vi "Test Report Contains Failed Test Result.vi"(8 "error in (no error)":errorcluster, 11 "Text Report Test in":refnum<class "Text Report Test.lvclass">) -> (0 "error out":errorcluster, 3 "Text Report Test out":refnum<class "Text Report Test.lvclass">)   [LabVIEW 2020, in "Text Report Test.lvclass"]
uses:
  Text Report Test.lvclass
  Test Doubles/Test Case Test Double/Methods.ctl
  Text Report Test.lvclass/Text Report Test.ctl
  Test Doubles/Test Case Test Double/Test Case Test Double.lvclass
  source/Plugins/Text Report/Text Report.lvclass
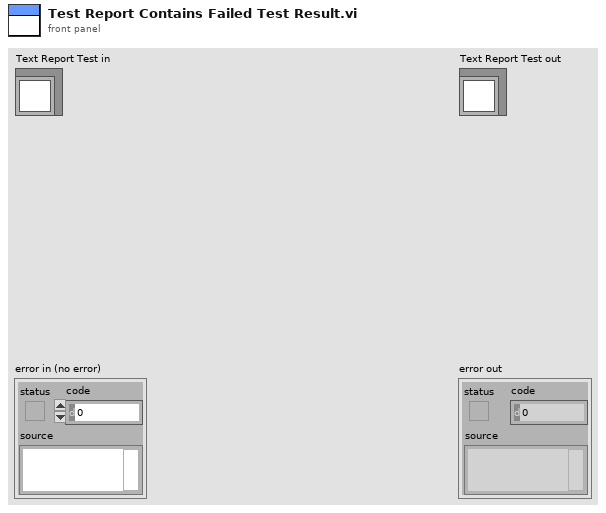
[diagram p1: front panel]
types:
  T1 = typedef "Test Case Test Double.lvclass/Methods.ctl" = enum16{"Test Failing Test.vi", "Test Passing Test.vi", "Test Error Test.vi", "Test Skip Test.vi", "Test Passing Pass If Test.vi", "Test Failing Pass If Test.vi", "Test Failing Fail If Test.vi", "Test Passing Fail If Test.vi", "Test Passing Pass If Error Test.vi", "Test Failing Pass If Error Test.vi", "Test Passing Fail If Error Test.vi", "Test Failing Fail If Error Test.vi", "Test Passing Pass If Equal Test.vi", "Test Failing Pass If Equal Test.vi", "Test Failing Fail If Equal Test.vi", "Test Passing Fail If Equal Test.vi", "Freezing Test.vi"}
  T2 = typedef "Result.lvlib/Result.ctl" = cluster{"Name":string, "Message":string, "Description":string, "Status":T3, "Result Type":T4, "Execution Time":dbl}
  T3 = typedef "Result.lvlib/Status.ctl" = enum16{"", "Passed", "Failed", "Error", "Skipped", "Setup Error", "Broken", "Teardown Error"}
  T4 = typedef "Result.lvlib/Type.ctl" = enum16{"Method", "Case", "Suite", "Pass", "Fail", "Skip", "Pass if", "Fail if", "Pass if Error", "Fail if Error", "Pass if Equal", "Fail if Equal"}
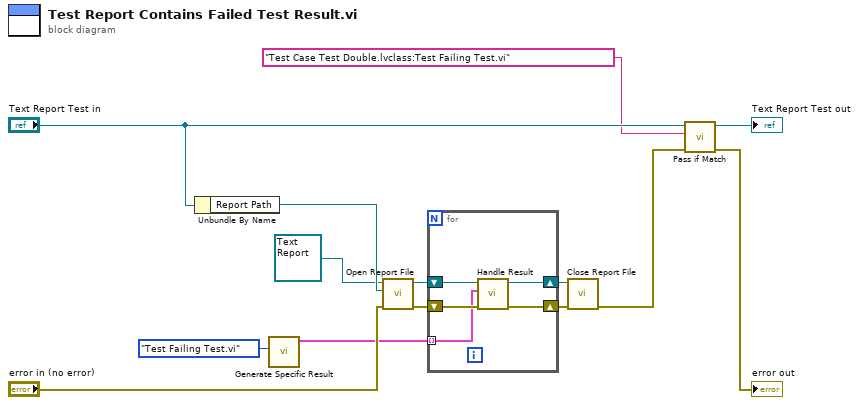
[diagram p0: block diagram]
diagram:
  n1 = Unbundle By Name("Text Report Test in") -> ("Report Path"=w13:path)
  n2 = call "Generate Specific Result.vi"("Test Method"=Methods."Test Failing Test.vi") -> ("Data"=w3:T2[])  [unwired: 9 in, 1 out]
  n3 = call-dynamic "Open Report File.vi"("error in (no error)"="error in (no error)", "Path"=w13, "Text Report In"=refnum<class "Text Report.lvclass"> refnum ("XML Report In")) -> ("error out"=w14:errorcluster, "Text Report Out"=w10:refnum<class "Text Report.lvclass">)  [unwired: 7 in]
  n4 = for {
    shift-right: [w18] -> w11
    shift-left: w14 -> [w19]
    shift-right: [w16] -> w9
    shift-left: w10 -> [w17]
    tunnel: w3 -> [w15] mode=indexing
    n5 = call-dynamic "Handle Result.vi"("error in (no error)"=w19, "Result"=w15, "Report in"=w17) -> ("error out"=w18:errorcluster, "Report out"=w16:refnum<class "Text Report.lvclass">)  [unwired: 7 in]
  }
  n6 = call-dynamic "Close Report File.vi"("error in (no error)"=w11, "Text Report In"=w9) -> ("error out"=w4:errorcluster)  [unwired: 9 in]
  n7 = call "Pass if Match.vi"("error in (no error)"=w4, "regular expression"="Test Case Test Double.lvclass:Test Failing Test.vi", "XML Report Test in"="Text Report Test in") -> ("error out"=→"error out":errorcluster, "XML Report Test out"=→"Text Report Test out":refnum<class "Text Report Test.lvclass">)  [unwired: 6 in, 1 out]
